vi "EXAMPLE_APPLICATION.vi"() -> ()   [LabVIEW 2017]
uses:
  DEF-SineSettings.ctl
  471e7864-20c3-404c-98e7-f175320ee992.vi
  29098ccc-a777-4c86-add4-ccc82f89efc3.vi
  42b5d3c3-b881-4cea-b812-ae5d7735da2d.vi
  dbaf8c0e-77fc-4e43-a2ad-cfefb2b50758.vi
  c4f9922d-01df-495a-9b54-5fd9be9e7843.vi
  TagDB/_Support/DataAccess/_NameCacher.vi
  TagDB/_Support/DataAccess/_datatypeChecker.vi
  TagDB/_Support/DataAccess/TagDB Ref to DVR.vi
  <vilib>/Utility/Data Type/Get Type Information.vi
  <vilib>/Utility/error.llb/Trim Whitespace.vi
  TagDB/_Support/Error/_[error50000]Invalid DB REF.vi
  TagDB/_Support/Error/_[error50002]Invalid DataType.vi
  TagDB/TagDB(DEV).lvlib
panel:
  in  "Model":bool
  out "Sine Settings":T1={"frequency"=10.0, "amplitude"=1.0, "phase"=0.0, "sampling info"={"Fs"=1000.0, "#s"=1000.0}} {"frequency" format="%0.2p"; "amplitude" format="%0.2p"; "phase" format="%.2p"; "sampling info"."Fs" format="%.2p"}
  out "Waveform Graph":waveform(dbl)(graph)
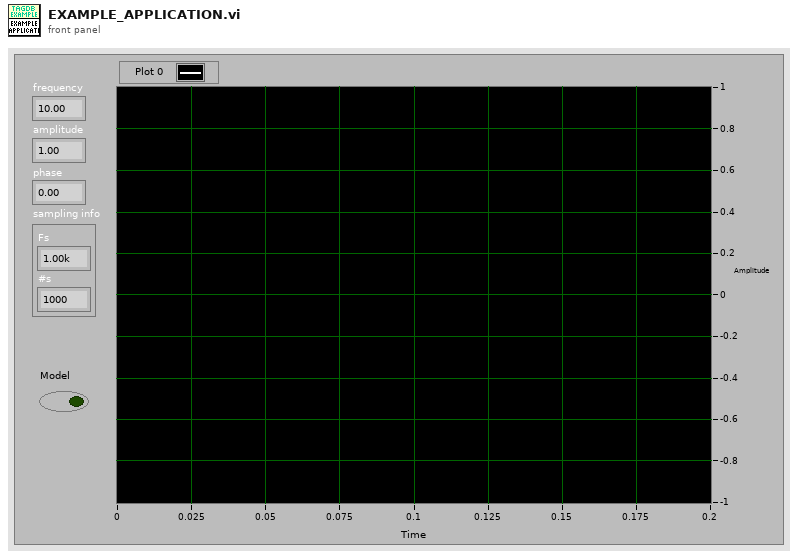
[diagram p1: front panel]
types:
  T1 = typedef "DEF-SineSettings.ctl" = cluster{"frequency":dbl, "amplitude":dbl, "phase":dbl, "sampling info":cluster{"Fs":dbl, "#s":dbl}}
  T2 = typedef "TagDB(DEV).lvlib/TagDB.ctl" = refnum<k1>
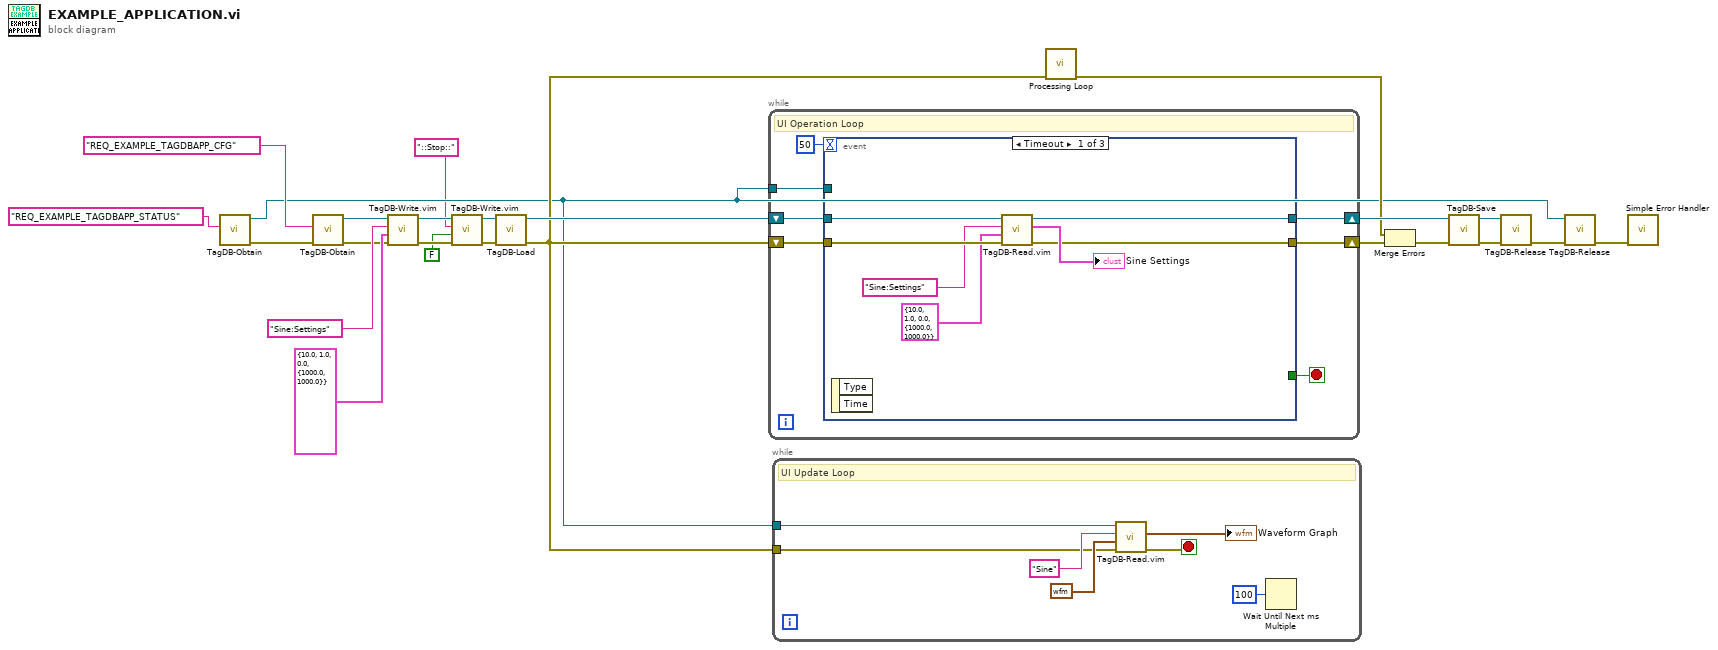
[diagram p0: block diagram]
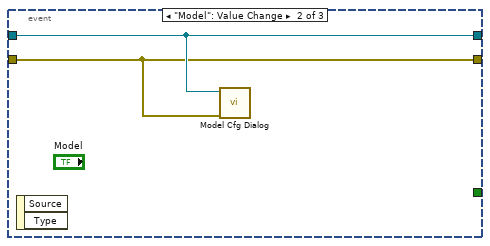
[diagram p2: hidden frame]
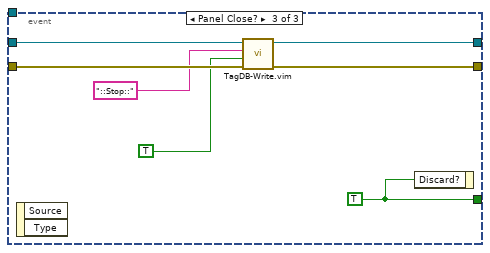
[diagram p3: hidden frame]
diagram:
  n1 = call "TagDB-Obtain.vi"("name (unnamed)"="REQ_EXAMPLE_TAGDBAPP_STATUS") -> ("error out"=w18:errorcluster, "TagDB"=w7:T2)  [unwired: 4 in, 1 out]
  n2 = call "TagDB-Obtain.vi"("error in (no error)"=w18, "name (unnamed)"="REQ_EXAMPLE_TAGDBAPP_CFG") -> ("error out"=w8:errorcluster, "TagDB"=w9:T2)  [unwired: 3 in, 1 out]
  n3 = call "TagDB-Write.vim"("error in (no error)"=w8, "Value"=T1 {"frequency"=10.0, "amplitude"=1.0, "phase"=0.0, "sampling info"={"Fs"=1000.0, "#s"=1000.0}} ("Sine Settings"), "name"="Sine:Settings", "TagDB"=w9) -> ("error out"=w6:errorcluster, "TagDB(dup)"=w3:T2)  [unwired: 5 in, 1 out]
  n4 = call "TagDB-Write.vim"("error in (no error)"=w6, "Value"=FALSE ("Reject New Tag(F)"), "name"="::Stop::", "TagDB"=w3) -> ("error out"=w5:errorcluster, "TagDB(dup)"=w4:T2)  [unwired: 5 in, 1 out]
  n5 = call "TagDB-Load.vi"("error in (no error)"=w5, "DB Ref"=w4) -> ("error out"=w14:errorcluster, "DB Ref(dup)"=w15:T2)  [unwired: 8 in]
  n6 = while {
    shift-right: [w28] -> w21
    shift-left: w15 -> [w29]
    shift-right: [w27] -> w20
    shift-left: w14 -> [w26]
    tunnel: w7 -> [w25]
    stop <- w31 stop-if-true
    # "UI Operation Loop"
    n7 = event shown="[0] Timeout" {
      selector: _ -> [_ _ _]
      dyn-events: _ -> [_ _ _]
      timeout: 50 -> [_ _ _]
      tunnel: [_ _ w47] -> w31
      tunnel: w29 -> [w38 w40 w46]
      tunnel: [w36 w40 w45] -> w28
      tunnel: [w32 w39 w43] -> w27
      tunnel: w26 -> [w37 w39 w44]
      tunnel: w25 -> [_ _ _]
      event Timeout {
        n8 = event-data() -> ()  [unwired: 1 in, 2 out]
        n9 = call "TagDB-Read.vim"("error in (no error)"=w37, "Type"=T1 {"frequency"=10.0, "amplitude"=1.0, "phase"=0.0, "sampling info"={"Fs"=1000.0, "#s"=1000.0}} ("Sine Settings"), "name"="Sine:Settings", "TagDB"=w38) -> ("error out"=w32:errorcluster, "Value"=→"Sine Settings":T1, "TagDB(dup)"=w36:T2)  [unwired: 2 in, 3 out]
      }
      event "Model": Value Change {
        n10 = event-data() -> ()  [unwired: 1 in, 2 out]
        n11 = call "Model Cfg Dialog.vi"("error in (no error)"=w39, "DB Ref"=w40) -> ()  [unwired: 9 in, 1 out]
      }
      event Panel Close? {
        w47 = TRUE
        n12 = event-data() -> ()  [unwired: 1 in, 2 out]
        n13 = call "TagDB-Write.vim"("error in (no error)"=w44, "Value"=TRUE, "name"="::Stop::", "TagDB"=w46) -> ("error out"=w43:errorcluster, "TagDB(dup)"=w45:T2)  [unwired: 5 in, 1 out]
        n14 = event-data ("Event Filter Node")("Discard?"=w47) -> ()  [unwired: 1 in, 1 out]
      }
    }
  }
  n15 = while {
    tunnel: w7 -> [w54]
    tunnel: w14 -> [w49]
    stop <- w53 stop-if-true
    # "UI Update Loop"
    n16 = call "TagDB-Read.vim"("error in (no error)"=w49, "Type"=waveform(dbl) {"t0"=timestamp(0 s since 1904-01-01), "dt"=1.0, "Y"=[]} ("signal out"), "name"="Sine", "TagDB"=w54) -> ("error out"=w53:errorcluster, "Value"=→"Waveform Graph":waveform(dbl))  [unwired: 2 in, 4 out]
    n17 = Wait Until Next ms Multiple(millisecond multiple=u32 100 ("milliseconds to wait")) -> ()  [unwired: 1 out]
  }
  n18 = call "Processing Loop.vi"("error in (no error)"=w14) -> ("error out"=w12:errorcluster)  [unwired: 10 in]
  n19 = Merge Errors(w12, w20) -> (w13:errorcluster)
  n20 = call "TagDB-Save.vi"("error in (no error)"=w13, "DB Ref"=w21) -> ("error out"=w22:errorcluster, "DB Ref(dup)"=w23:T2)  [unwired: 8 in]
  n21 = call "TagDB-Release.vi"("error in (no error)"=w22, "TagDB"=w23) -> ("error out"=w17:errorcluster)  [unwired: 9 in]
  n22 = call "TagDB-Release.vi"("error in (no error)"=w17, "TagDB"=w7) -> ("error out"=w16:errorcluster)  [unwired: 9 in]
  n23 = call <vilib>:"Simple Error Handler.vi"("error in (no error)"=w16) -> ()  [unwired: 4 in, 5 out]
